vi "子界面-查看某框-只读穿透图模式.vi"(0 "框号":dbl format="%#_13g", 1 "框组":T3(array[cluster]), 2 "临界Z值":i32, 4 "临界面积百分比值":dbl, 5 "预先配置的灰度阈值":dbl, 6 "穿透图原始路径":path, 7 "部位信息":string[](array[string])=["", "34.500000", "32.500000", "1121", "34", "54.955926", "分层类", "不合格", ""], 12 "产品规格":cluster{"产品长度（周长）（mm）":dbl, "产品宽度（母线长）（mm）":dbl}) -> (14 "弥散类检测结果":string[][](table), 19 "分层类检测结果":string[][](table))   [LabVIEW 2018]
uses:
  <vilib>/vision/NI_Vision_Development_Module.lvlib
panel:
  out "Pixel Measurements":i32[](array[ring])=[0, 1, 2, 23, 24, 0, 1, 48] items=["Bounding Rect Width", "Bounding Rect Height", "Area"]
  in  "Tab Control":T1
  out "?":T2(plugin-control)
  out "Threshold Image":T2(plugin-control)
  out "Threshold Image":T2(plugin-control)
  in  "格式字符串 3":string="%f"
  in  "分隔符（'\\'代码显示） 2":string="\t"
  out "弥散和分层临界灰度值":i64
  out "弥散缺陷个数":i32
  out "分层缺陷个数":i32
  out "合格？ 弥散类":string="fencengThreshold"
  out "合格？分层类":string="fencengThreshold"
  in  "stop":bool caption="停止"
  out "弥散测量结果":dbl[][](array[numeric]) format="%.2f"
  out "?":string
  out "面积 (pixels)":i32
  in  "格式字符串 2":string="%f"
  in  "分隔符（'\\'代码显示）":string="\t"
  out "分层测量结果":dbl[][](array[numeric]) format="%.2f"
  out "缺陷初步分类的临界值":sgl format="%#.3f"
  # "所选区域信息"
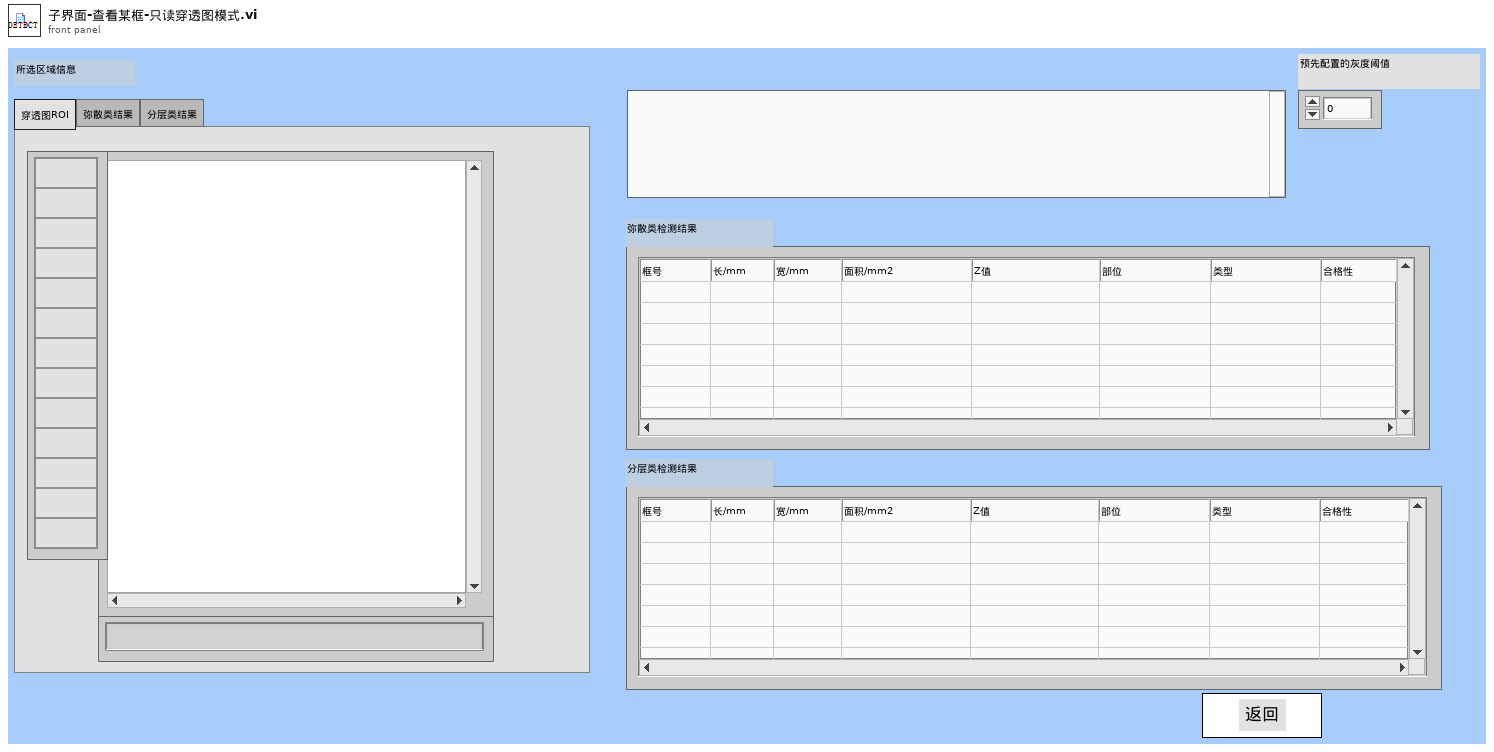
[diagram p1: front panel]
types:
  T1 = typedef "控件2.ctl" = enum32{"穿透图ROI", "弥散类结果", "分层类结果"}
  T2 = typedef "IMAQ Image.ctl" = refnum<image>
  T3 = cluster{"Global Rectangle":i32[], "Contours":cluster{"Contour Type":u32, "ROI Type":u32, "Points":i32[]}[]}[]
  T4 = typedef "Image Type" = u32
  T5 = cluster{"Global Rectangle":i32[], "Contours":cluster{"Contour Type":u32, "ROI Type":u32, "Points":i32[]}[]}
  T6 = typedef "Particle Parameters" = i32
  T7 = cluster{"Measurement Parameter":T6, "Range Lower Value":dbl, "Range Upper Value":dbl, "Range":bool, "Measurement Type":bool}[]
  T8 = cluster{"histogram":u32[], "Minimal Value":sgl, "Maximal Value":sgl, "Starting Value":sgl, "Interval Width":sgl, "Mean Value":sgl, "Standard  Variation":sgl, "Area (pixels)":i32}
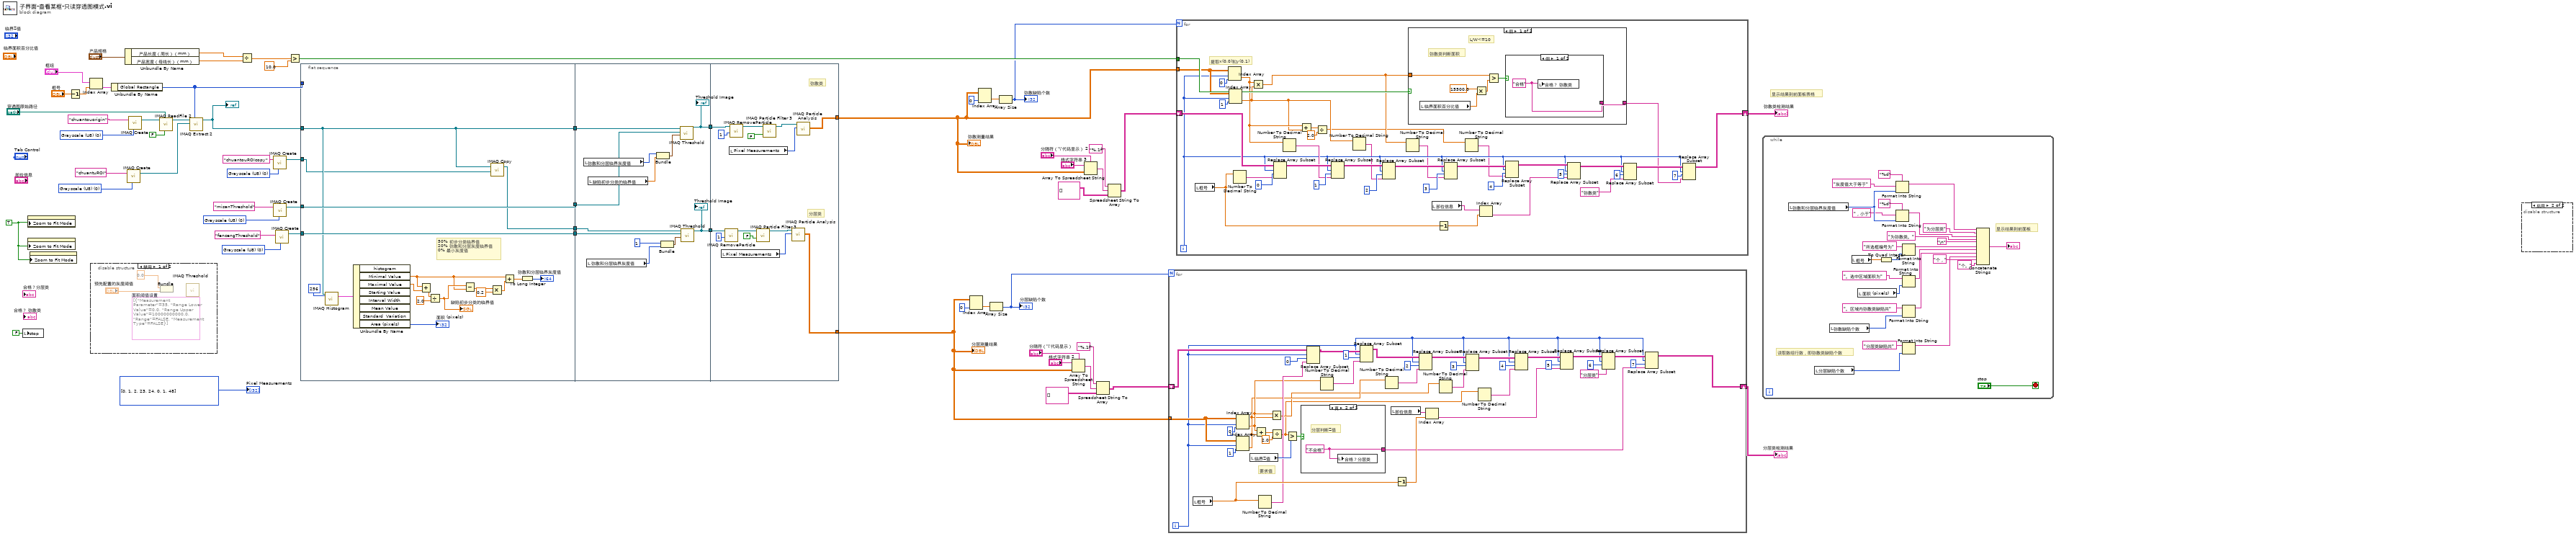
[diagram p0: block diagram]
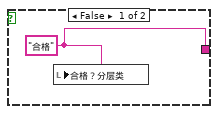
[diagram p3: hidden frame]
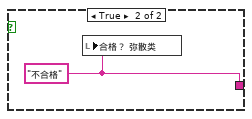
[diagram p4: hidden frame]
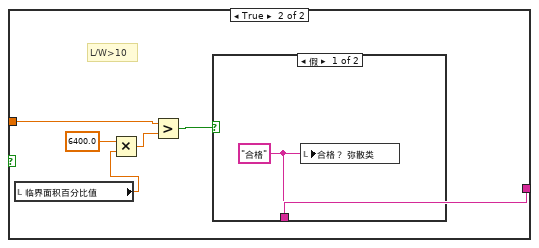
[diagram p5: hidden frame]
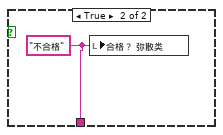
[diagram p6: hidden frame]
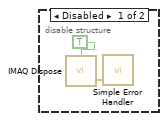
[diagram p7: hidden frame]
diagram:
  w1 = T4 0 items=["Grayscale (U8)", "Grayscale (I16)", "Grayscale (SGL)", "Complex (CSG)", "RGB (U32)", "HSL (U32)", "RGB (U64)", "Grayscale (U16)"] ("Image Type")
  w5 = TRUE ("Zoom to Fit Mode")
  w37 = T4 0 items=["Grayscale (U8)", "Grayscale (I16)", "Grayscale (SGL)", "Complex (CSG)", "RGB (U32)", "HSL (U32)", "RGB (U64)", "Grayscale (U16)"] ("Image Type")
  w38 = T4 0 items=["Grayscale (U8)", "Grayscale (I16)", "Grayscale (SGL)", "Complex (CSG)", "RGB (U32)", "HSL (U32)", "RGB (U64)", "Grayscale (U16)"] ("Image Type")
  w41 = T4 0 items=["Grayscale (U8)", "Grayscale (I16)", "Grayscale (SGL)", "Complex (CSG)", "RGB (U32)", "HSL (U32)", "RGB (U64)", "Grayscale (U16)"] ("Image Type")
  w25 = i32[] [0, 1, 2, 23, 24, 0, 1, 48] items=["Bounding Rect Width", "Bounding Rect Height", "Area"] ("Pixel Measurements")
  w56 = T4 0 items=["Grayscale (U8)", "Grayscale (I16)", "Grayscale (SGL)", "Complex (CSG)", "RGB (U32)", "HSL (U32)", "RGB (U64)", "Grayscale (U16)"] ("Image Type")
  # "显示结果到前面板表格"
  n1 = local write "stop"(FALSE ("stop")) -> ()
  n2 = property class="ImageControl"("Zoom to Fit Mode"=w5) -> ()  [unwired: 2 in, 2 out]
  n3 = property class="ImageControl"("Zoom to Fit Mode"=w5) -> ()  [unwired: 2 in, 2 out]
  n4 = property class="ImageControl"("Zoom to Fit Mode"=w5) -> ()  [unwired: 2 in, 2 out]
  n5 = Decrement(x="框号") -> (x-1=w58:dbl)
  n6 = Index Array(array="框组", index=w58) -> (element=w59:T5)
  n7 = disable-structure shown="禁用" {
    frame Disabled {
      (unwired) T7 [{"Measurement Parameter"=35, "Range Lower Value"=0.0, "Range Upper Value"=10000000000.0, "Range"=FALSE, "Measurement Type"=FALSE}]  # 面积阈值设置
      n8 = Bundle(0.0, "预先配置的灰度阈值"="预先配置的灰度阈值") -> ()  [unwired: 1 in, 1 out]
      n9 = call "IMAQ Threshold"() -> ()  [unwired: 6 in, 6 out]
    }
    frame Enabled {
    }
  }
  n10 = Unbundle By Name(w59) -> ("Global Rectangle"=w32:i32[])
  n11 = Unbundle By Name("产品规格") -> ("产品长度（周长）（mm）"=w49:dbl, "产品宽度（母线长）（mm）"=w48:dbl)
  n12 = call "IMAQ Create"("Image Name"="chuantuROI", "Image Type"=w41) -> ("New Image"=w40:T2)  [unwired: 3 in, 1 out]
  n13 = call "IMAQ Create"("Image Name"="chuantouorigin", "Image Type"=w56) -> ("New Image"=w43:T2)  [unwired: 3 in, 1 out]
  n14 = call "IMAQ ReadFile 2"("Use File Path Image Type"=FALSE, "File Path"="穿透图原始路径", "Image"=w43) -> ("Image Out"=w44:T2)  [unwired: 4 in, 4 out]
  n15 = call "IMAQ Extract 2"("Optional Rectangle"=w32, "Image Dst"=w40, "Image Src"=w44) -> ("Image Dst Out"=w7:T2)  [unwired: 7 in, 1 out]
  "?" <- w7
  n16 = Divide(x=w49, y=w48) -> (x/y=w52:dbl)
  n17 = call "IMAQ Create"("Image Name"="chuantouROIcopy", "Image Type"=w1) -> ("New Image"=w3:T2)  [unwired: 3 in, 1 out]
  n18 = call "IMAQ Create"("Image Name"="misanThreshold", "Image Type"=w37) -> ("New Image"=w30:T2)  [unwired: 3 in, 1 out]
  n19 = call "IMAQ Create"("Image Name"="fencengThreshold", "Image Type"=w38) -> ("New Image"=w29:T2)  [unwired: 3 in, 1 out]
  n20 = Greater?(x=w52, y=10.0) -> (0:w47:bool)
  n21 = flat-sequence {
    tunnel: [w81] -> w31
    tunnel: [w80] -> w28
    tunnel: [w66] -> w6
    tunnel: [w65] -> w4
    tunnel: w32 -> [_]
    tunnel: w30 -> [w81]
    tunnel: w29 -> [w80]
    tunnel: w7 -> [w66]
    tunnel: w3 -> [w64]
    tunnel: w31 -> [w93]
    tunnel: w28 -> [w92]
    tunnel: [w84] -> w27
    tunnel: [w85] -> w26
    tunnel: w6 -> [w86]
    tunnel: w4 -> [w83]
    tunnel: [w94] -> w10
    tunnel: [w105] -> w18
    tunnel: w27 -> [w100]
    tunnel: w26 -> [w97]
    frame #0 {
      # "50% 初步分类临界值\n20% 弥散和分层灰度临界值\n0% 最小灰度值"
      n22 = call "IMAQ Histogram"("Number of Classes"=256, "Image"=w66) -> ("Histogram Report"=w78:T8)  [unwired: 8 in, 1 out]
      n23 = Unbundle By Name(w78) -> ("Minimal Value"=w68:sgl, "Maximal Value"=w74:sgl, "Area (pixels)"=→"面积 (pixels)":i32)  [unwired: 5 out]
      n24 = Add(x=w68, y=w74) -> (x+y=w73:sgl)
      n25 = Divide(x=w73, y=sgl 2.0) -> (x/y=w72:sgl)
      "缺陷初步分类的临界值" <- w72
      n26 = Subtract(x=w72, y=w68) -> (x-y=w70:sgl)
      n27 = Multiply(x=w70, y=0.2) -> (x*y=w69:dbl)
      n28 = call "IMAQ Copy"("Image Dst"=w64, "Image Src"=w66) -> ("Image Dst Out"=w65:T2)  [unwired: 4 in, 1 out]
      n29 = Add(x=w68, y=w69) -> (x+y=w67:dbl)
      n30 = To Long Integer(number=w67) -> (32bit integer=→"弥散和分层临界灰度值":i32)
    }
    frame #1 {
      n31 = local read "弥散和分层临界灰度值"() -> (w82:i64)
      n32 = local read "弥散和分层临界灰度值"() -> (w88:i64)
      n33 = local read "缺陷初步分类的临界值"() -> (w90:sgl)
      n34 = Bundle("弥散和分层临界灰度值"=w82, "缺陷初步分类的临界值"=w90) -> (w91:cluster{"弥散和分层临界灰度值":i64, "缺陷初步分类的临界值":sgl})  [unwired: 1 in]
      n35 = Bundle(1, "弥散和分层临界灰度值"=w88) -> (w87:cluster{i32, "弥散和分层临界灰度值":i64})  [unwired: 1 in]
      n36 = call "IMAQ Threshold"("Range"=w91, "Image Dst"=w93, "Image Src"=w86) -> ("Image Dst Out"=w85:T2)  [unwired: 3 in, 5 out]
      "Threshold Image" <- w85
      n37 = call "IMAQ Threshold"("Range"=w87, "Image Dst"=w92, "Image Src"=w83) -> ("Image Dst Out"=w84:T2)  [unwired: 3 in, 5 out]
      "Threshold Image" <- w84
    }
    frame #2 {
      # "分层类"
      # "弥散类"
      n38 = local read "Pixel Measurements"() -> (w102:i32[])
      n39 = call "IMAQ RemoveParticle"("Number of Erosion"=1, "Image Src"=w100) -> ("Image Dst Out"=w101:T2)  [unwired: 8 in, 1 out]
      n40 = local read "Pixel Measurements"() -> (w103:i32[])
      n41 = call "IMAQ RemoveParticle"("Number of Erosion"=1, "Image Src"=w97) -> ("Image Dst Out"=w98:T2)  [unwired: 8 in, 1 out]
      n42 = call "IMAQ Particle Filter 3"("Image Src"=w101, "Keep/Remove Particles (F)"=FALSE) -> ("Image Dst Out"=w104:T2)  [unwired: 11 in, 2 out]
      n43 = call "IMAQ Particle Filter 3"("Image Src"=w98, "Keep/Remove Particles (F)"=FALSE) -> ("Image Dst Out"=w95:T2)  [unwired: 11 in, 2 out]
      n44 = call "IMAQ Particle Analysis"("Pixel Measurements"=w102, "Image"=w104) -> ("Particle Measurements (Pixels)"=w105:dbl[][])  [unwired: 4 in, 5 out]
      n45 = call "IMAQ Particle Analysis"("Pixel Measurements"=w103, "Image"=w95) -> ("Particle Measurements (Pixels)"=w94:dbl[][])  [unwired: 4 in, 5 out]
    }
  }
  n46 = Index Array(array=w18, index (col)=0 ("禁用的索引 (列)")) -> (element=w36:dbl[])  [unwired: 1 in]
  n47 = Index Array(array=w10, index (col)=0 ("禁用的索引 (列)")) -> (element=w34:dbl[])  [unwired: 1 in]
  n48 = Array Size(array=w36) -> (size(s)=w24:i32)
  "分层缺陷个数" <- w24
  n49 = Array Size(array=w34) -> (size(s)=w46:i32)
  "弥散缺陷个数" <- w46
  n50 = Array To Spreadsheet String(delimiter (Tab)="分隔符（'\\'代码显示）", array=w18, 3:"格式字符串 2") -> (spreadsheet string=w21:string)
  n51 = Array To Spreadsheet String(delimiter (Tab)="分隔符（'\\'代码显示） 2", array=w10, 3:"格式字符串 3") -> (spreadsheet string=w13:string)
  n52 = Spreadsheet String To Array(format string="%.1f", spreadsheet string=w21, array type (2D Dbl)=string[][] [] ("Array")) -> (array=w17:string[][])  [unwired: 1 in]
  n53 = Spreadsheet String To Array(format string="%.1f", spreadsheet string=w13, array type (2D Dbl)=string[][] [] ("Array")) -> (array=w9:string[][])  [unwired: 1 in]
  n54 = for {
    N: w24 -> [_]
    tunnel: w18 -> [w139]
    shift-right: [w117] -> w16
    shift-left: w17 -> [w128]
    i -> [w112]
    # "要求值"
    n55 = local read "框号"() -> (w137:dbl)
    n56 = Index Array(array=w139, index (row)=w112, index (col)=0 ("禁用的索引 (列)")) -> (element=w116:dbl)
    n57 = Index Array(array=w139, index (row)=w112, index (col)=1 ("禁用的索引 (列)")) -> (element=w115:dbl)
    n58 = local read "临界Z值"() -> (w145:i32)
    n59 = Add(x=w116, y=w115) -> (x+y=w146:dbl)
    n60 = Number To Decimal String(number=w137) -> (decimal integer string=w129:string)  [unwired: 1 in]
    n61 = Multiply(x=w116, y=w115) -> (x*y=w114:dbl)
    n62 = Divide(x=w146, y=2.0) -> (x/y=w111:dbl)
    n63 = Greater?(x=w111, y=w145) -> (0:w147:bool)
    n64 = case shown="真" w147 {
      tunnel: [w148 w149] -> w108
      frame False {
        w148 = "合格" ("合格？")
        n65 = local write "合格？分层类"(w148) -> ()
      }
      frame True {
        w149 = "不合格" ("合格？")
        # "分层判断Z值"
        n66 = local write "合格？分层类"(w149) -> ()
      }
    }
    n67 = Replace Array Subset(array=w128, new element=w129, index (row)=w112, index (col)=0 ("索引 (列)")) -> (w127:string[][])
    n68 = Number To Decimal String(number=w116) -> (decimal integer string=w126:string)  [unwired: 1 in]
    n69 = Replace Array Subset(array=w127, new element=w126, index (row)=w112, index (col)=1 ("索引 (列)")) -> (w124:string[][])
    n70 = Number To Decimal String(number=w115) -> (decimal integer string=w125:string)  [unwired: 1 in]
    n71 = local read "部位信息"() -> (w141:string[])
    n72 = Decrement(x=w137) -> (x-1=w140:dbl)
    n73 = Replace Array Subset(array=w124, new element=w125, index (row)=w112, index (col)=2 ("索引 (列)")) -> (w123:string[][])
    n74 = Index Array(array=w141, index=w140) -> (element=w110:string)
    n75 = Number To Decimal String(number=w114) -> (decimal integer string=w122:string)  [unwired: 1 in]
    n76 = Replace Array Subset(array=w123, new element=w122, index (row)=w112, index (col)=3 ("索引 (列)")) -> (w121:string[][])
    n77 = Number To Decimal String(number=w111) -> (decimal integer string=w113:string)  [unwired: 1 in]
    n78 = Replace Array Subset(array=w121, new element=w113, index (row)=w112, index (col)=4 ("索引 (列)")) -> (w120:string[][])
    n79 = Replace Array Subset(array=w120, new element=w110, index (row)=w112, index (col)=5 ("索引 (列)")) -> (w119:string[][])
    n80 = Replace Array Subset(array=w119, new element="分层类" ("新元素/子数组"), index (row)=w112, index (col)=6 ("索引 (列)")) -> (w118:string[][])
    n81 = Replace Array Subset(array=w118, new element=w108, index (row)=w112, index (col)=7 ("索引 (列)")) -> (w117:string[][])
  }
  "分层类检测结果" <- w16
  n82 = for {
    N: w46 -> [_]
    tunnel: w47 -> [w188]
    tunnel: w10 -> [w187]
    shift-right: [w167] -> w8
    shift-left: w9 -> [w175]
    i -> [w165]
    # "提取x(0,0)和y(0,1)"
    n83 = local read "框号"() -> (w153:dbl)
    n84 = Index Array(array=w187, index (row)=w165, index (col)=0 ("禁用的索引 (列)")) -> (element=w159:dbl)
    n85 = Index Array(array=w187, index (row)=w165, index (col)=1 ("禁用的索引 (列)")) -> (element=w158:dbl)
    n86 = Number To Decimal String(number=w153) -> (decimal integer string=w176:string)  [unwired: 1 in]
    n87 = Multiply(x=w159, y=w158) -> (x*y=w163:dbl)
    n88 = Replace Array Subset(array=w175, new element=w176, index (row)=w165, index (col)=0 ("索引 (列)")) -> (w174:string[][])
    n89 = Number To Decimal String(number=w159) -> (decimal integer string=w166:string)  [unwired: 1 in]
    n90 = Add(x=w159, y=w158) -> (x+y=w161:dbl)
    n91 = Divide(x=w161, y=2.0) -> (x/y=w157:dbl)
    n92 = Replace Array Subset(array=w174, new element=w166, index (row)=w165, index (col)=1 ("索引 (列)")) -> (w173:string[][])
    n93 = Number To Decimal String(number=w158) -> (decimal integer string=w164:string)  [unwired: 1 in]
    n94 = Replace Array Subset(array=w173, new element=w164, index (row)=w165, index (col)=2 ("索引 (列)")) -> (w172:string[][])
    n95 = Number To Decimal String(number=w163) -> (decimal integer string=w162:string)  [unwired: 1 in]
    n96 = case shown="假" w188 {
      tunnel: w163 -> [w194 w202]
      tunnel: [w192 w200] -> w150
      frame False {
        # "弥散类判断面积"
        # "L/W<=10"
        n97 = local read "临界面积百分比值"() -> (w190:dbl)
        n98 = Multiply(x=15500.0, y=w190) -> (x*y=w189:dbl)
        n99 = Greater?(x=w194, y=w189) -> (0:w193:bool)
        n100 = case shown="假" w193 {
          tunnel: [w195 w196] -> w192
          frame False {
            w195 = "合格" ("合格？")
            n101 = local write "合格？ 弥散类"(w195) -> ()
          }
          frame True {
            w196 = "不合格" ("合格？")
            n102 = local write "合格？ 弥散类"(w196) -> ()
          }
        }
      }
      frame True {
        # "L/W>10"
        n103 = local read "临界面积百分比值"() -> (w197:dbl)
        n104 = Multiply(x=6400.0, y=w197) -> (x*y=w199:dbl)
        n105 = Greater?(x=w202, y=w199) -> (0:w201:bool)
        n106 = case shown="假" w201 {
          tunnel: [w203 w204] -> w200
          frame False {
            w203 = "合格" ("合格？")
            n107 = local write "合格？ 弥散类"(w203) -> ()
          }
          frame True {
            w204 = "不合格" ("合格？")
            n108 = local write "合格？ 弥散类"(w204) -> ()
          }
        }
      }
    }
    n109 = local read "部位信息"() -> (w155:string[])
    n110 = Decrement(x=w153) -> (x-1=w154:dbl)
    n111 = Replace Array Subset(array=w172, new element=w162, index (row)=w165, index (col)=3 ("索引 (列)")) -> (w171:string[][])
    n112 = Number To Decimal String(number=w157) -> (decimal integer string=w156:string)  [unwired: 1 in]
    n113 = Index Array(array=w155, index=w154) -> (element=w152:string)
    n114 = Replace Array Subset(array=w171, new element=w156, index (row)=w165, index (col)=4 ("索引 (列)")) -> (w170:string[][])
    n115 = Replace Array Subset(array=w170, new element=w152, index (row)=w165, index (col)=5 ("索引 (列)")) -> (w169:string[][])
    n116 = Replace Array Subset(array=w169, new element="弥散类" ("新元素/子数组"), index (row)=w165, index (col)=6 ("索引 (列)")) -> (w168:string[][])
    n117 = Replace Array Subset(array=w168, new element=w150, index (row)=w165, index (col)=7 ("索引 (列)")) -> (w167:string[][])
  }
  "弥散类检测结果" <- w8
  n118 = while {
    stop <- "stop" stop-if-true
    # "显示结果到前面板"
    # "读取数组行数，即弥散类缺陷个数"
    n119 = local read "弥散和分层临界灰度值"() -> (w231:i64)
    n120 = local read "分层缺陷个数"() -> (w206:i32)
    n121 = local read "弥散缺陷个数"() -> (w205:i32)
    n122 = local read "框号"() -> (w222:dbl)
    n123 = local read "面积 (pixels)"() -> (w225:i32)
    n124 = To Quad Integer(1:w222) -> (0:w223:i64)
    n125 = Format Into String(format string="%d" ("格式字符串"), initial string="灰度值大于等于" ("初始字符串"), w231) -> (resulting string=w227:string)  [unwired: 1 in, 1 out]
    n126 = Format Into String(format string="%d" ("格式字符串"), initial string="，小于" ("初始字符串"), w231) -> (resulting string=w226:string)  [unwired: 1 in, 1 out]
    n127 = Format Into String(initial string="所选框编号为" ("初始字符串"), w223) -> (resulting string=w221:string)  [unwired: 2 in, 1 out]
    n128 = Format Into String(initial string="。选中区域面积为" ("字符串"), w225) -> (resulting string=w228:string)  [unwired: 2 in, 1 out]
    n129 = Format Into String(initial string="。区域内弥散类缺陷共" ("初始字符串"), w205) -> (resulting string=w229:string)  [unwired: 2 in, 1 out]
    n130 = Format Into String(initial string="分层类缺陷共" ("初始字符串"), w206) -> (resulting string=w230:string)  [unwired: 2 in, 1 out]
    n131 = Concatenate Strings(w227, "为分层类" ("初始字符串"), w226, "为弥散类。" ("初始字符串"), "\n", w221, w228, w229, "个，" ("字符串"), w230, "个。" ("字符串")) -> (→"?":string)
  }
  n132 = disable-structure shown="启用" {
    frame Disabled {
      n133 = call "IMAQ Dispose"("All Images? (No)"=TRUE) -> ("error out"=w233:errorcluster)  [unwired: 5 in]
      n134 = call <vilib>:"Simple Error Handler.vi"("error in (no error)"=w233) -> ()  [unwired: 4 in, 5 out]
    }
    frame Enabled {
    }
  }
  "分层测量结果" <- w18
  "弥散测量结果" <- w10
  "Pixel Measurements" <- w25
